vi "send_BrakeForce.vi"(4 "Counter":i32, 5 "200/freq":i32=1, 6 "Active":bool, 7 "CAN ID":u32=657 format="%x", 8 "Message":cluster{"Brake force [bar]":dbl} {"Brake force [bar]" scale=0.0..2000.0}, 11 "CAN frame":T1[](array[typedef]) {"Data" format="%.0x"; "ArbitrationId" format="%.0x"; "Timestamp" format="%<%I:%M:%S%3u %p\n%m/%d/%Y>T"}) -> (3 "CAN frame out":T1[](array[typedef]) {"Data" format="%.0x"; "ArbitrationId" format="%.0x"; "Timestamp" format="%<%I:%M:%S%3u %p\n%m/%d/%Y>T"})   [LabVIEW 2017]
uses:
  <vilib>/nican/nican.llb/CanFrameTimed.ctl
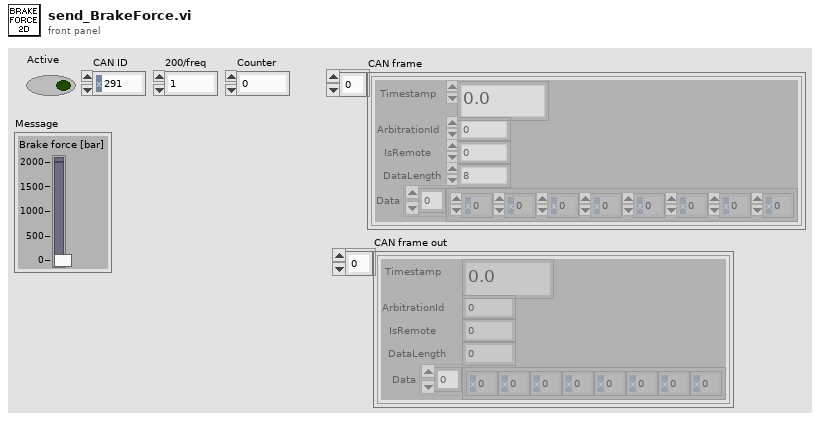
[diagram p1: front panel]
types:
  T1 = typedef "CanFrameTimed.ctl" = cluster{"Timestamp":dbl, "ArbitrationId":u32, "IsRemote":u8, "DataLength":u8, "Data":u8[]}
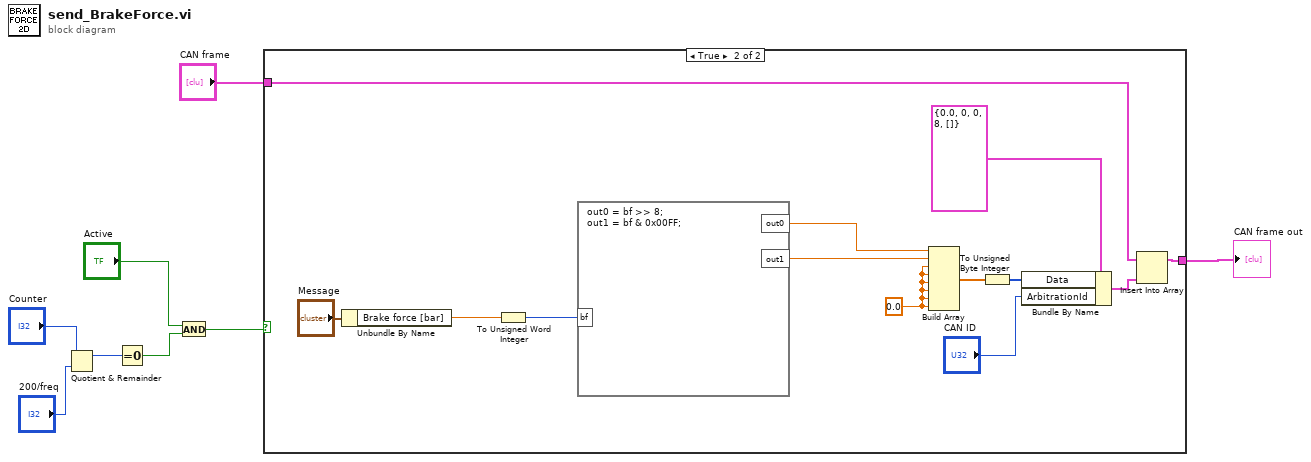
[diagram p0: block diagram]
diagram:
  n1 = Quotient & Remainder(x="Counter", y="200/freq") -> (x-y*floor(x/y)=w5:i32)  [unwired: 1 out]
  n2 = Equal To 0?(x=w5) -> (x = 0?=w3:bool)
  n3 = And(x="Active", y=w3) -> (x .and. y?=w2:bool)
  n4 = case shown="True" w2 {
    tunnel: "CAN frame" -> [w9 w19]
    tunnel: [w9 w17] -> w7
    frame False {
    }
    frame True {
      w12 = 0.0 ("element")
      n5 = Unbundle By Name("Message") -> ("Brake force [bar]"=w11:dbl)
      n6 = To Unsigned Word Integer(number=w11) -> (unsigned 16bit integer=w10:u16)
      n7 = formula code="out0 = bf >> 8;\nout1 = bf & 0x00FF;"("bf"=w10) -> ("out0"=w14:dbl, "out1"=w13:dbl)
      n8 = Build Array(w14, w13, w12, w12, w12, w12, w12, w12) -> (w22:dbl[])
      n9 = To Unsigned Byte Integer(number=w22) -> (unsigned 8bit integer=w21:u8[])
      n10 = Bundle By Name(cluster=T1 {"Timestamp"=0.0, "ArbitrationId"=0, "IsRemote"=0, "DataLength"=8, "Data"=[]} ("CAN frame"), "Data"=w21, "ArbitrationId"="CAN ID") -> (w18:T1)
      n11 = Insert Into Array(array=w19, new element=w18) -> (w17:T1[])  [unwired: 1 in]
    }
  }
  "CAN frame out" <- w7
